vi "displayImage.vi"(8 "error in (no error)":errorcluster, 10 "Path":path, 11 "ImageStreamViewer in":refnum<class "ImageStreamViewer.lvclass">) -> (0 "error out":errorcluster, 3 "ImageStreamViewer out":refnum<class "ImageStreamViewer.lvclass">)   [LabVIEW 2009, in "Views.lvlib" / "Camera.lvlib" / "ImageStreamViewer.lvclass"]
uses:
  ImageStreamViewer.lvclass
  ImageStreamViewer.lvclass/ImageStreamViewer.ctl
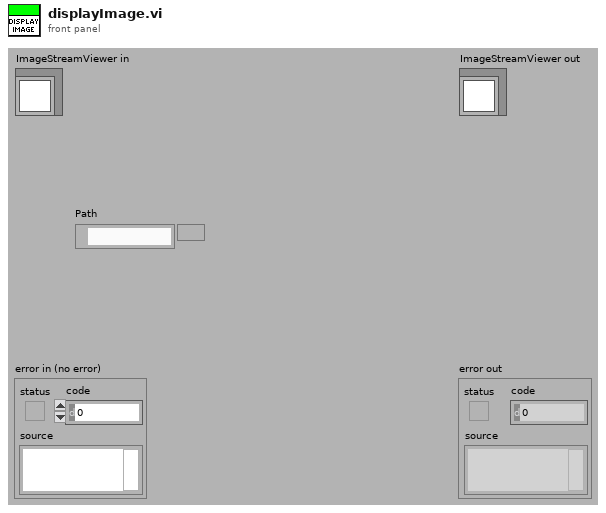
[diagram p1: front panel]
types:
  T1 = typedef "IMAQ Image.ctl" = refnum<image>
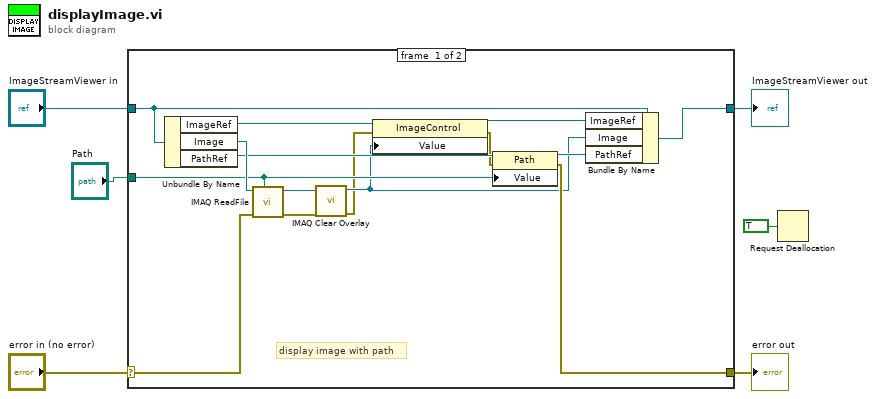
[diagram p0: block diagram]
diagram:
  n1 = case shown="No Error" "error in (no error)" {
    selector: "error in (no error)" -> [w20 w23]
    tunnel: [w13 w23] -> w5
    tunnel: [w17 w22] -> w3
    tunnel: "ImageStreamViewer in" -> [w18 w22]
    tunnel: "Path" -> [w15 _]
    frame #0 {
      # "display image with path"
      n2 = Unbundle By Name(w18) -> ("ImageRef"=w7:refnum<vi>, "Image"=w21:T1, "PathRef"=w16:refnum<vi>)
      n3 = call "IMAQ ReadFile"("File Path"=w15, "error in (no error)"=w20, "Image"=w21) -> ("error out"=w9:errorcluster, "Image Out"=w11:T1)  [unwired: 4 in, 3 out]
      n4 = call "IMAQ Clear Overlay"("error in (no error)"=w9, "Image"=w11) -> ("error out"=w8:errorcluster, "Image Out"=w10:T1)  [unwired: 8 in]
      n5 = property class="ImageControl"(reference=w7, error in=w8, "Value"=w10) -> (reference out=w19:refnum<vi>, error out=w14:errorcluster)
      n6 = property class="Path"(reference=w16, error in=w14, "Value"=w15) -> (reference out=w12:refnum<vi>, error out=w13:errorcluster)
      n7 = Bundle By Name(cluster=w18, "ImageRef"=w19, "Image"=w10, "PathRef"=w12) -> (w17:refnum<class "ImageStreamViewer.lvclass">)
    }
    frame #1 {
    }
  }
  "error out" <- w5
  "ImageStreamViewer out" <- w3
  n8 = Request Deallocation(TRUE ("flag")) -> ()
